vi "Unevenly Sampled Signal Spectrum.vi"(0 "XTime":dbl[](array[numeric]) format="%.2f", 1 "X":dbl[](array[numeric]) format="%.2f") -> (2 "Power Spectrum FFT {X} Frequency":dbl[](array[numeric]) format="%.2f", 3 "Power Spectrum FFT {X}":dbl[](array[numeric]) format="%.2f", 4 "error":i32)   [LabVIEW 2009]
doc: "Calculates the power spectrum of a signal that is unevenly spaced in time."
uses:
  <vilib>/Analysis/baseanly.llb/Real Dot Product.vi
  <vilib>/Analysis/NI_AALBase.lvlib
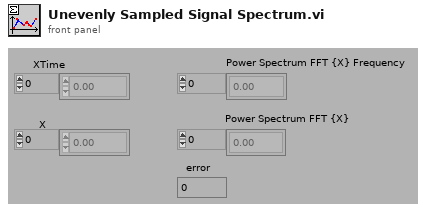
[diagram p1: front panel]
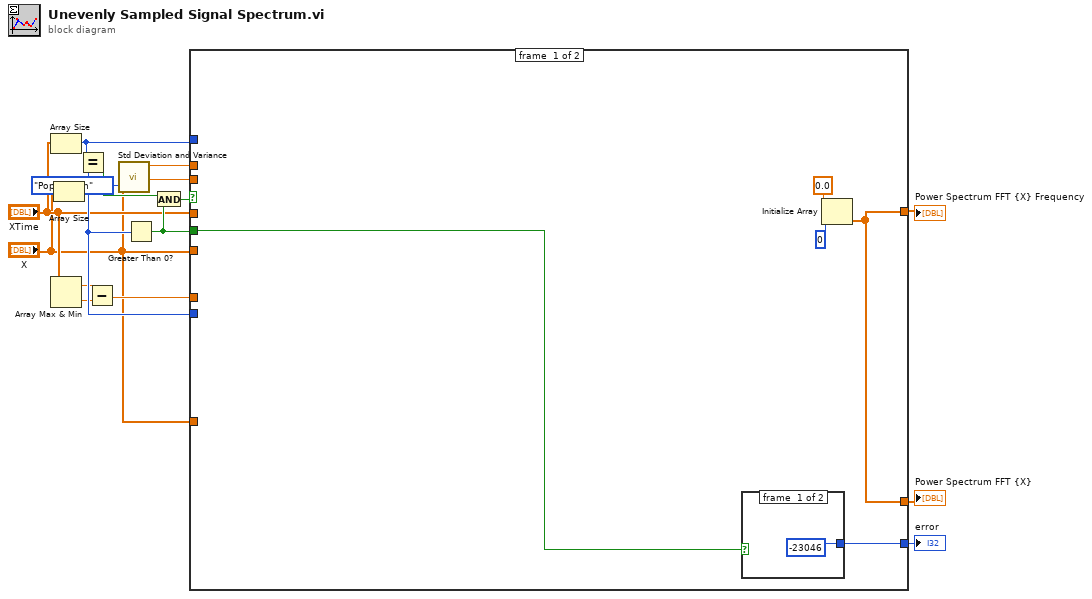
[diagram p0: block diagram]
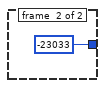
[diagram p2: hidden frame]
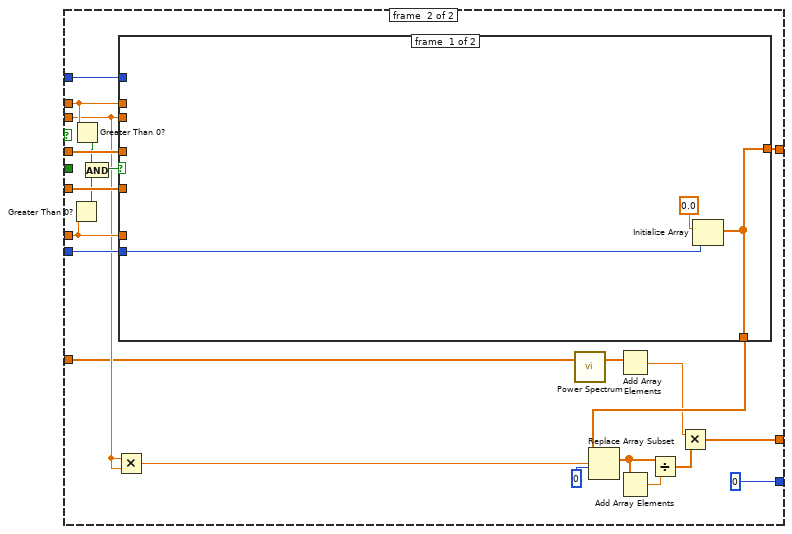
[diagram p3: hidden frame]
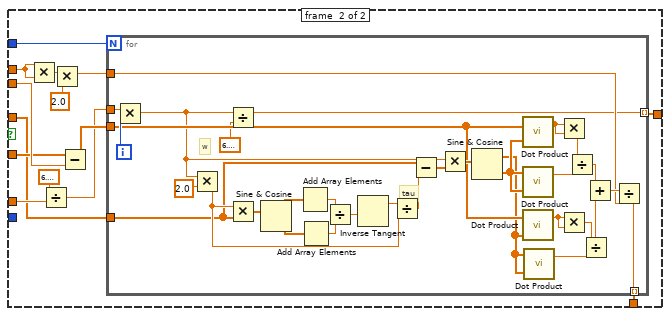
[diagram p4: hidden frame]
diagram:
  n1 = Array Size(array="XTime") -> (size(s)=w13:i32)
  n2 = Array Max & Min(array="XTime") -> (max value=w6:dbl, min value=w5:dbl)  [unwired: 2 out]
  n3 = Array Size(array="X") -> (size(s)=w8:i32)
  n4 = Equal?(x=w13, y=w8) -> (x = y?=w12:bool)
  n5 = Subtract(x=w6, y=w5) -> (x-y=w4:dbl)
  n6 = call "Std Deviation and Variance.vi"("X"="X", "Weighting (Sample)"=enum16{"Sample", "Population"}."Population") -> ("mean"=w3:dbl, "standard deviation"=w9:dbl)  [unwired: 1 out]
  n7 = Greater Than 0?(x=w8) -> (x > 0?=w10:bool)
  n8 = And(x=w12, y=w10) -> (x .and. y?=w11:bool)
  n9 = case shown="True" w11 {
    tunnel: w13 -> [_ w42]
    tunnel: "X" -> [_ w45]
    tunnel: "XTime" -> [_ w44]
    tunnel: [w19 w28] -> w15
    tunnel: [w19 w24] -> w16
    tunnel: [w17 0] -> w14
    tunnel: w10 -> [w18 _]
    tunnel: w9 -> [_ w41]
    tunnel: w3 -> [_ w33]
    tunnel: w8 -> [_ w40]
    tunnel: w4 -> [_ w39]
    tunnel: "X" -> [_ w27]
    frame #0 {
      n10 = case shown="True" w18 {
        tunnel: [-23046 -23033] -> w17
        frame #0 {
        }
        frame #1 {
        }
      }
      n11 = Initialize Array(0.0, 0) -> (w19:dbl[])
    }
    frame #1 {
      n12 = Greater Than 0?(x=w39) -> (x > 0?=w37:bool)
      n13 = Greater Than 0?(x=w41) -> (x > 0?=w38:bool)
      n14 = And(x=w38, y=w37) -> (x .and. y?=w36:bool)
      n15 = Multiply(x=w33, y=w33) -> (x*y=w32:dbl)
      n16 = case shown="True" w36 {
        tunnel: w33 -> [_ w62]
        tunnel: w41 -> [_ w61]
        tunnel: w42 -> [_ w52]
        tunnel: [w46 w51] -> w35
        tunnel: w44 -> [_ w50]
        tunnel: w45 -> [_ w55]
        tunnel: w40 -> [w47 _]
        tunnel: w39 -> [_ w53]
        tunnel: [w46 w49] -> w24
        frame #0 {
          n17 = Initialize Array(0.0, w47) -> (w46:dbl[])
        }
        frame #1 {
          n18 = Multiply(x=w61, y=w61) -> (x*y=w59:dbl)
          n19 = Divide(x=6.283185307179586, y=w53) -> (x/y=w56:dbl)
          n20 = Multiply(x=w59, y=2.0) -> (x*y=w57:dbl)
          n21 = Subtract(x=w55, y=w62) -> (x-y=w60:dbl[])
          n22 = for {
            N: w52 -> [_]
            tunnel: [w63] -> w49 mode=indexing
            tunnel: w50 -> [w84]
            tunnel: w60 -> [w76]
            tunnel: w57 -> [w68]
            tunnel: [w67] -> w51 mode=indexing
            tunnel: w56 -> [w66]
            i -> [w94]
            # "w"
            # "tau"
            n23 = Multiply(x=w66, y=w94) -> (x*y=w65:dbl)
            n24 = Multiply(x=w65, y=2.0) -> (x*y=w85:dbl)
            n25 = Divide(x=w65, y=6.283185307179586) -> (x/y=w63:dbl)
            n26 = Multiply(x=w85, y=w84) -> (x*y=w92:dbl[])
            n27 = Sine & Cosine(0:w92) -> (1:w91:dbl[], 2:w90:dbl[])
            n28 = Add Array Elements(numeric array=w91) -> (sum=w89:dbl)
            n29 = Add Array Elements(numeric array=w90) -> (sum=w88:dbl)
            n30 = Divide(x=w89, y=w88) -> (x/y=w87:dbl)
            n31 = Inverse Tangent(1:w87) -> (0:w86:dbl)
            n32 = Divide(x=w86, y=w85) -> (x/y=w83:dbl)
            n33 = Subtract(x=w84, y=w83) -> (x-y=w82:dbl[])
            n34 = Multiply(x=w65, y=w82) -> (x*y=w81:dbl[])
            n35 = Sine & Cosine(0:w81) -> (1:w74:dbl[], 2:w79:dbl[])
            n36 = call-poly <vilib>:"Dot Product.vi"("Y Vector"=w79, "X Vector"=w76) -> ("X * Y"=w80:dbl)  [unwired: 1 out]
            n37 = call-poly <vilib>:"Dot Product.vi"("Y Vector"=w79, "X Vector"=w79) -> ("X * Y"=w78:dbl)  [unwired: 1 out]
            n38 = call-poly <vilib>:"Dot Product.vi"("Y Vector"=w74, "X Vector"=w76) -> ("X * Y"=w75:dbl)  [unwired: 1 out]
            n39 = call-poly <vilib>:"Dot Product.vi"("Y Vector"=w74, "X Vector"=w74) -> ("X * Y"=w72:dbl)  [unwired: 1 out]
            n40 = Multiply(x=w80, y=w80) -> (x*y=w77:dbl)
            n41 = Multiply(x=w75, y=w75) -> (x*y=w73:dbl)
            n42 = Divide(x=w77, y=w78) -> (x/y=w71:dbl)
            n43 = Divide(x=w73, y=w72) -> (x/y=w70:dbl)
            n44 = Add(x=w71, y=w70) -> (x+y=w69:dbl)
            n45 = Divide(x=w69, y=w68) -> (x/y=w67:dbl)
          }
        }
      }
      n46 = call "Power Spectrum.vi"("X"=w27) -> ("Power Spectrum"=w26:dbl[])  [unwired: 1 out]
      n47 = Replace Array Subset(array=w35, new element=w32, index=0) -> (w31:dbl[])
      n48 = Add Array Elements(numeric array=w26) -> (sum=w25:dbl)
      n49 = Add Array Elements(numeric array=w31) -> (sum=w30:dbl)
      n50 = Divide(x=w31, y=w30) -> (x/y=w29:dbl[])
      n51 = Multiply(x=w25, y=w29) -> (x*y=w28:dbl[])
    }
  }
  "Power Spectrum FFT {X}" <- w15
  "error" <- w14
  "Power Spectrum FFT {X} Frequency" <- w16
